vi "ntitled 1 (2).vi"() -> ()   [LabVIEW 2020]
panel:
  out "Numeric 4":dbl
  in  "Numeric 3":dbl
  in  "Numeric 2":dbl
  in  "Numeric":dbl
  out "Meter":dbl(knob) scale=0.0..10.0
  in  "Tank":dbl(slide) scale=0.0..10.0
  out "Thermometer":dbl(slide) scale=0.0..100.0
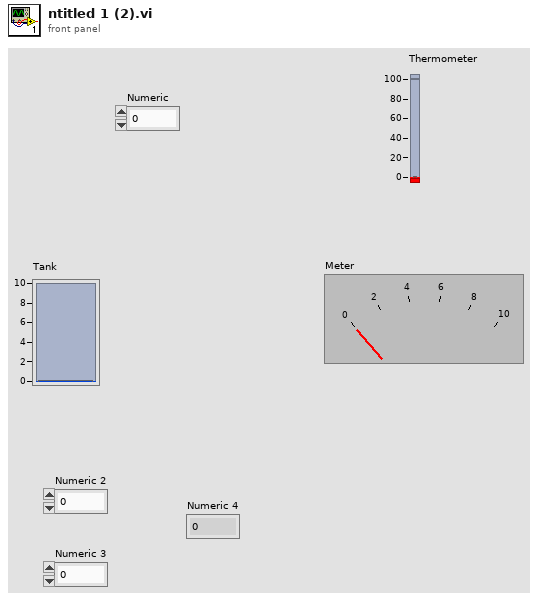
[diagram p1: front panel]
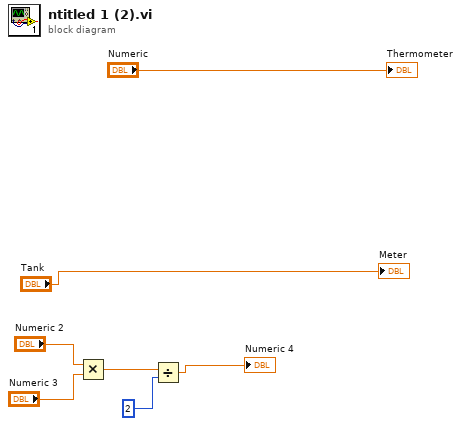
[diagram p0: block diagram]
diagram:
  n1 = Multiply(x="Numeric 2", y="Numeric 3") -> (x*y=w3:dbl)
  n2 = Divide(x=w3, y=2) -> (x/y=→"Numeric 4":dbl)
  "Thermometer" <- "Numeric"
  "Meter" <- "Tank"
